vi "Help.Page.Get.vi"(11 "GUID":string) -> (2 "HTML File":string="PIDs.html", 3 "Main CHM File":string="Diagnostics.chm")   [LabVIEW 2019, in "Diagnostics Addon System Explorer.lvlib"]
uses:
  Diagnostics Addon System Explorer.lvlib
  Addon Shared/SubVIs/Constants.vi
  Addon Shared/Diagnostics Addon Shared.lvlib
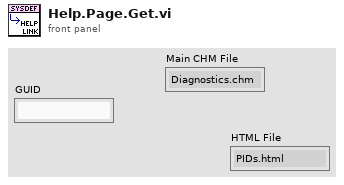
[diagram p1: front panel]
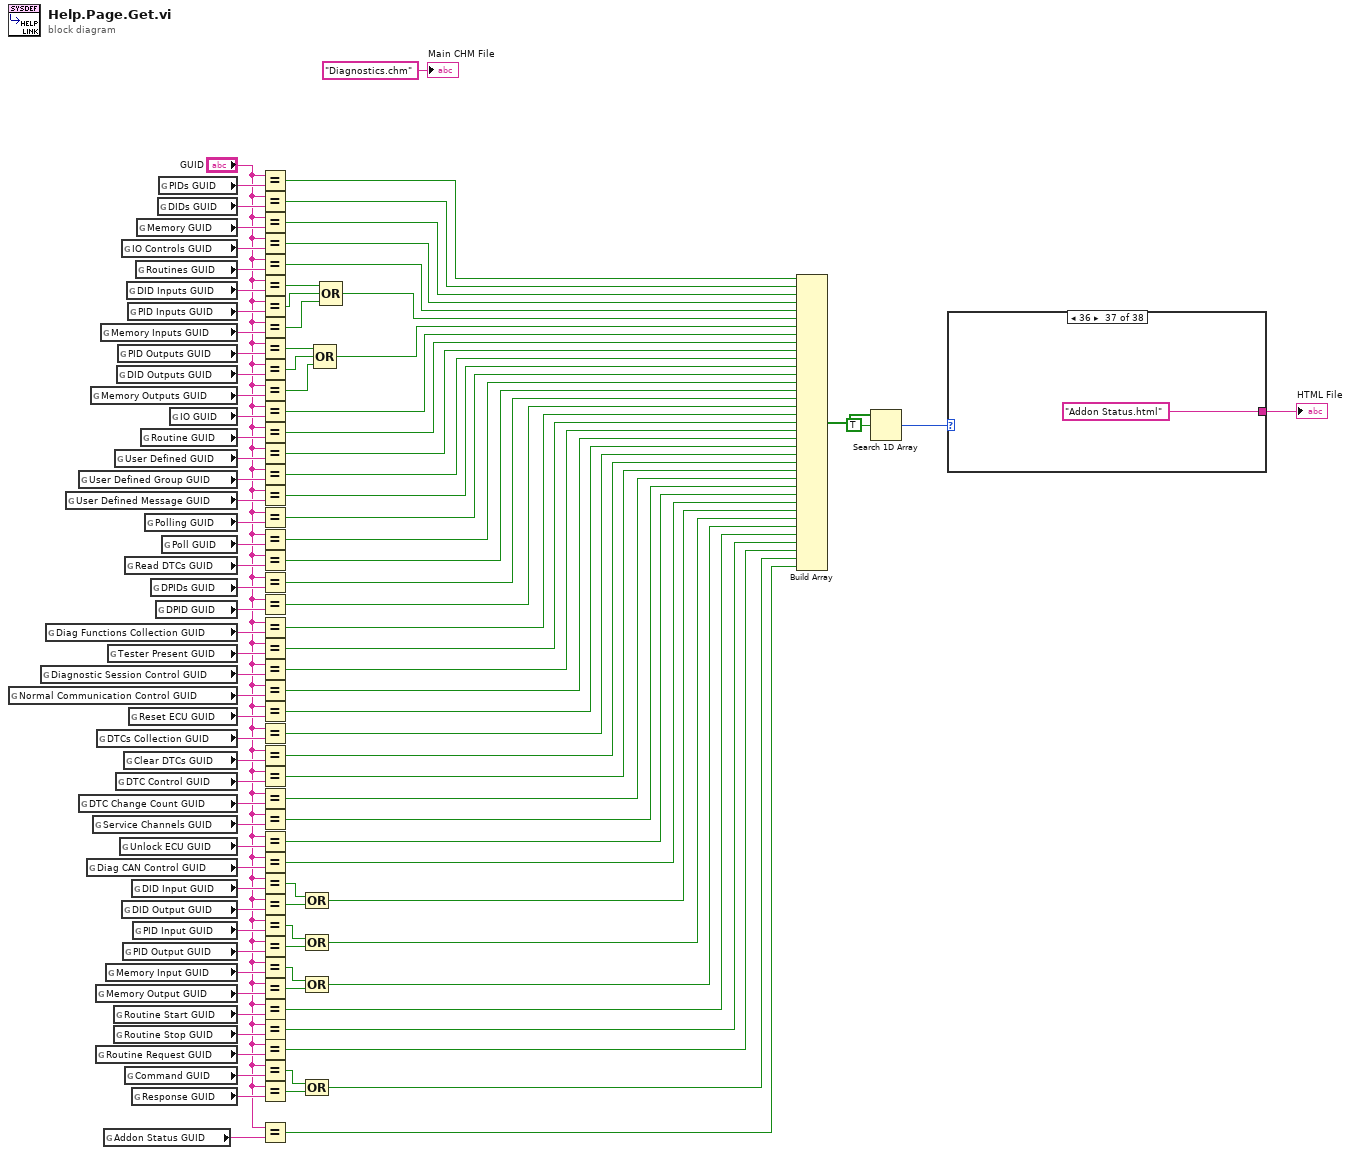
[diagram p0: block diagram]
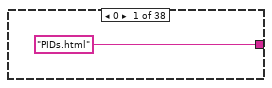
[diagram p2: hidden frame]
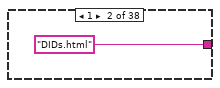
[diagram p3: hidden frame]
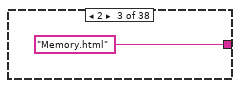
[diagram p4: hidden frame]
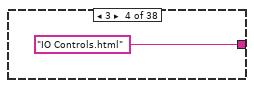
[diagram p5: hidden frame]
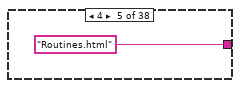
[diagram p6: hidden frame]
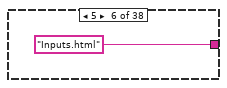
[diagram p7: hidden frame]
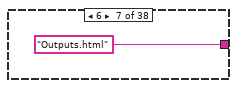
[diagram p8: hidden frame]
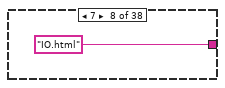
[diagram p9: hidden frame]
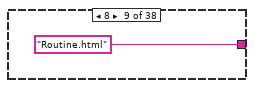
[diagram p10: hidden frame]
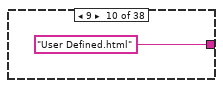
[diagram p11: hidden frame]
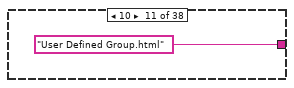
[diagram p12: hidden frame]
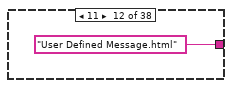
[diagram p13: hidden frame]
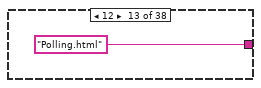
[diagram p14: hidden frame]
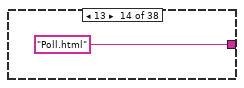
[diagram p15: hidden frame]
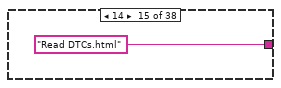
[diagram p16: hidden frame]
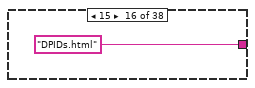
[diagram p17: hidden frame]
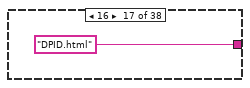
[diagram p18: hidden frame]
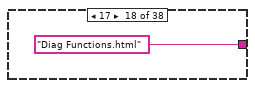
[diagram p19: hidden frame]
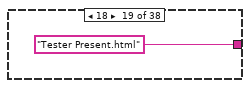
[diagram p20: hidden frame]
diagram:
  n1 = global read "Constants.vi" "Normal Communication Control GUID"() -> (w47:string)
  n2 = global read "Constants.vi" "Diagnostic Session Control GUID"() -> (w49:string)
  n3 = global read "Constants.vi" "Diag Functions Collection GUID"() -> (w45:string)
  n4 = global read "Constants.vi" "User Defined Message GUID"() -> (w81:string)
  n5 = global read "Constants.vi" "User Defined Group GUID"() -> (w82:string)
  n6 = global read "Constants.vi" "DTC Change Count GUID"() -> (w53:string)
  n7 = global read "Constants.vi" "Diag CAN Control GUID"() -> (w31:string)
  n8 = global read "Constants.vi" "Memory Outputs GUID"() -> (w86:string)
  n9 = global read "Constants.vi" "Service Channels GUID"() -> (w35:string)
  n10 = global read "Constants.vi" "Memory Output GUID"() -> (w24:string)
  n11 = global read "Constants.vi" "Routine Request GUID"() -> (w23:string)
  n12 = global read "Constants.vi" "DTCs Collection GUID"() -> (w50:string)
  n13 = global read "Constants.vi" "Memory Inputs GUID"() -> (w95:string)
  n14 = global read "Constants.vi" "Addon Status GUID"() -> (w3:string)
  n15 = global read "Constants.vi" "Memory Input GUID"() -> (w25:string)
  n16 = global read "Constants.vi" "Tester Present GUID"() -> (w46:string)
  n17 = global read "Constants.vi" "Routine Start GUID"() -> (w21:string)
  n18 = global read "Constants.vi" "Routine Stop GUID"() -> (w22:string)
  n19 = global read "Constants.vi" "User Defined GUID"() -> (w80:string)
  n20 = global read "Constants.vi" "DTC Control GUID"() -> (w52:string)
  n21 = global read "Constants.vi" "DID Outputs GUID"() -> (w87:string)
  n22 = global read "Constants.vi" "PID Outputs GUID"() -> (w96:string)
  n23 = global read "Constants.vi" "Unlock ECU GUID"() -> (w33:string)
  n24 = global read "Constants.vi" "IO Controls GUID"() -> (w98:string)
  n25 = global read "Constants.vi" "DID Output GUID"() -> (w28:string)
  n26 = global read "Constants.vi" "PID Output GUID"() -> (w26:string)
  n27 = global read "Constants.vi" "Clear DTCs GUID"() -> (w51:string)
  n28 = global read "Constants.vi" "Read DTCs GUID"() -> (w59:string)
  n29 = global read "Constants.vi" "Command GUID"() -> (w8:string)
  n30 = global read "Constants.vi" "DID Inputs GUID"() -> (w94:string)
  n31 = global read "Constants.vi" "PID Inputs GUID"() -> (w93:string)
  n32 = global read "Constants.vi" "Reset ECU GUID"() -> (w48:string)
  n33 = global read "Constants.vi" "DID Input GUID"() -> (w29:string)
  n34 = global read "Constants.vi" "Response GUID"() -> (w7:string)
  n35 = global read "Constants.vi" "PID Input GUID"() -> (w27:string)
  n36 = global read "Constants.vi" "Routines GUID"() -> (w97:string)
  n37 = global read "Constants.vi" "Memory GUID"() -> (w102:string)
  n38 = global read "Constants.vi" "Routine GUID"() -> (w84:string)
  n39 = global read "Constants.vi" "Polling GUID"() -> (w64:string)
  n40 = global read "Constants.vi" "DPIDs GUID"() -> (w57:string)
  n41 = global read "Constants.vi" "DPID GUID"() -> (w55:string)
  n42 = global read "Constants.vi" "DIDs GUID"() -> (w101:string)
  n43 = global read "Constants.vi" "PIDs GUID"() -> (w100:string)
  n44 = global read "Constants.vi" "Poll GUID"() -> (w62:string)
  n45 = global read "Constants.vi" "IO GUID"() -> (w83:string)
  n46 = Equal?(x="GUID", y=w100) -> (x = y?=w66:bool)
  n47 = Equal?(x="GUID", y=w101) -> (x = y?=w79:bool)
  n48 = Equal?(x="GUID", y=w102) -> (x = y?=w78:bool)
  n49 = Equal?(x="GUID", y=w98) -> (x = y?=w77:bool)
  n50 = Equal?(x="GUID", y=w97) -> (x = y?=w76:bool)
  n51 = Equal?(x="GUID", y=w94) -> (x = y?=w92:bool)
  n52 = Equal?(x="GUID", y=w93) -> (x = y?=w91:bool)
  n53 = Equal?(x="GUID", y=w95) -> (x = y?=w90:bool)
  n54 = Equal?(x="GUID", y=w96) -> (x = y?=w85:bool)
  n55 = Equal?(x="GUID", y=w87) -> (x = y?=w88:bool)
  n56 = Equal?(x="GUID", y=w86) -> (x = y?=w89:bool)
  n57 = Equal?(x="GUID", y=w83) -> (x = y?=w73:bool)
  n58 = Equal?(x="GUID", y=w84) -> (x = y?=w72:bool)
  n59 = Equal?(x="GUID", y=w80) -> (x = y?=w71:bool)
  n60 = Equal?(x="GUID", y=w82) -> (x = y?=w70:bool)
  n61 = Equal?(x="GUID", y=w81) -> (x = y?=w69:bool)
  n62 = Equal?(x="GUID", y=w64) -> (x = y?=w63:bool)
  n63 = Equal?(x="GUID", y=w62) -> (x = y?=w61:bool)
  n64 = Equal?(x="GUID", y=w59) -> (x = y?=w58:bool)
  n65 = Equal?(x="GUID", y=w57) -> (x = y?=w56:bool)
  n66 = Equal?(x="GUID", y=w55) -> (x = y?=w54:bool)
  n67 = Equal?(x="GUID", y=w45) -> (x = y?=w44:bool)
  n68 = Equal?(x="GUID", y=w46) -> (x = y?=w43:bool)
  n69 = Equal?(x="GUID", y=w49) -> (x = y?=w42:bool)
  n70 = Equal?(x="GUID", y=w47) -> (x = y?=w41:bool)
  n71 = Equal?(x="GUID", y=w48) -> (x = y?=w40:bool)
  n72 = Equal?(x="GUID", y=w50) -> (x = y?=w39:bool)
  n73 = Equal?(x="GUID", y=w51) -> (x = y?=w38:bool)
  n74 = Equal?(x="GUID", y=w52) -> (x = y?=w37:bool)
  n75 = Equal?(x="GUID", y=w53) -> (x = y?=w36:bool)
  n76 = Equal?(x="GUID", y=w35) -> (x = y?=w34:bool)
  n77 = Equal?(x="GUID", y=w33) -> (x = y?=w32:bool)
  n78 = Equal?(x="GUID", y=w31) -> (x = y?=w30:bool)
  n79 = Equal?(x="GUID", y=w29) -> (x = y?=w19:bool)
  n80 = Equal?(x="GUID", y=w28) -> (x = y?=w20:bool)
  n81 = Equal?(x="GUID", y=w27) -> (x = y?=w14:bool)
  n82 = Equal?(x="GUID", y=w26) -> (x = y?=w17:bool)
  n83 = Equal?(x="GUID", y=w25) -> (x = y?=w15:bool)
  n84 = Equal?(x="GUID", y=w24) -> (x = y?=w16:bool)
  n85 = Equal?(x="GUID", y=w21) -> (x = y?=w11:bool)
  n86 = Equal?(x="GUID", y=w22) -> (x = y?=w10:bool)
  n87 = Equal?(x="GUID", y=w23) -> (x = y?=w9:bool)
  n88 = Equal?(x="GUID", y=w8) -> (x = y?=w5:bool)
  n89 = Equal?(x="GUID", y=w7) -> (x = y?=w6:bool)
  n90 = Equal?(x="GUID", y=w3) -> (x = y?=w1:bool)
  n91 = Compound Arithmetic op=OR(w19, w20) -> (w18:bool)
  n92 = Compound Arithmetic op=OR(w14, w17) -> (w13:bool)
  n93 = Compound Arithmetic op=OR(w15, w16) -> (w12:bool)
  n94 = Compound Arithmetic op=OR(w5, w6) -> (w4:bool)
  n95 = Compound Arithmetic op=OR(w85, w88, w89) -> (w74:bool)
  n96 = Compound Arithmetic op=OR(w92, w91, w90) -> (w75:bool)
  n97 = Build Array(w66, w79, w78, w77, w76, w75, w74, w73, w72, w71, w70, w69, w63, w61, w58, w56, w54, w44, w43, w42, w41, w40, w39, w38, w37, w36, w34, w32, w30, w18, w13, w12, w11, w10, w9, w4, w1) -> (w68:bool[])
  n98 = Search 1D Array(1D array=w68, element=TRUE) -> (index of element=w65:i32)  [unwired: 1 in]
  n99 = case shown="36" w65 {
    tunnel: ["PIDs.html" ("HTML File") "DIDs.html" ("HTML File") "Memory.html" ("HTML File") "IO Controls.html" ("HTML File") "Routines.html" ("HTML File") "Inputs.html" ("HTML File") "Outputs.html" ("HTML File") "IO.html" ("HTML File") "Routine.html" ("HTML File") "User Defined.html" ("HTML File") "User Defined Group.html" ("HTML File") "User Defined Message.html" ("HTML File") "Polling.html" ("HTML File") "Poll.html" ("HTML File") "Read DTCs.html" ("HTML File") "DPIDs.html" ("HTML File") "DPID.html" ("HTML File") "Diag Functions.html" ("HTML File") "Tester Present.html" ("HTML File") "Diag Session Control.html" ("HTML File") "Communication Control.html" ("HTML File") "ECU Reset.html" ("HTML File") "DTCs Collection.html" ("HTML File") "Clear DTCs.html" ("HTML File") "Control DTCs.html" ("HTML File") "DTC Change Count.html" ("HTML File") "Service Channels.html" ("HTML File") "Unlock ECU.html" ("HTML File") "Diag CAN Control.html" ("HTML File") "DID ID.html" ("HTML File") "PID ID.html" ("HTML File") "Memory ID.html" ("HTML File") "Start Routine.html" ("HTML File") "Stop Routine.html" ("HTML File") "Request Routine.html" ("HTML File") "Frame.html" ("HTML File") "Addon Status.html" ("HTML File") "MainPage_Diag.html" ("HTML File")] -> w99
    frame 0 {
    }
    frame 1 {
    }
    frame 2 {
    }
    frame 3 {
    }
    frame 4 {
    }
    frame 5 {
    }
    frame 6 {
    }
    frame 7 {
    }
    frame 8 {
    }
    frame 9 {
    }
    frame 10 {
    }
    frame 11 {
    }
    frame 12 {
    }
    frame 13 {
    }
    frame 14 {
    }
    frame 15 {
    }
    frame 16 {
    }
    frame 17 {
    }
    frame 18 {
    }
    frame 19 {
    }
    frame 20 {
    }
    frame 21 {
    }
    frame 22 {
    }
    frame 23 {
    }
    frame 24 {
    }
    frame 25 {
    }
    frame 26 {
    }
    frame 27 {
    }
    frame 28 {
    }
    frame 29 {
    }
    frame 30 {
    }
    frame 31 {
    }
    frame 32 {
    }
    frame 33 {
    }
    frame 34 {
    }
    frame 35 {
    }
    frame 36 {
    }
    frame Default {
    }
  }
  "HTML File" <- w99
  "Main CHM File" <- "Diagnostics.chm" ("Main CHM File")
